vi "IsHotGoalDB.vi"(7 "Timeout (ms)":u32, 8 "error in":errorcluster, 9 "DBHot?":string="Boolean", 10 "DBFinished?":string="Boolean", 11 "DBStart":string="Boolean") -> (0 "error out":errorcluster, 1 "TimedOut?":bool, 2 "Hot?":bool, 3 "ElapsedTime":u32)   [LabVIEW 2015]
doc: "IsHotGoalDB determines whether or not the goal is hot. Image processing is done on the laptop (through the DB).\n-DBStart: the name of the DB boolean control that starts image processing. IsHotGoalDB writes to this to signal the DB to start.\n-DBFinished?: the name of the DB boolean indicator that indicates when the DB is done processing.\n-DBHot?: the name of the DB boolean indicator that indicates whether the goal is hot."
panel:
  in  "milliseconds to wait":u32=20
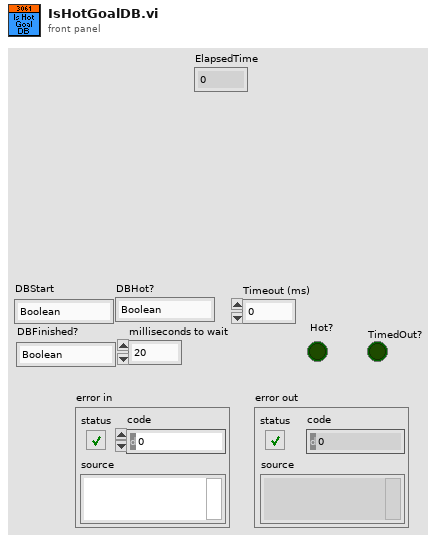
[diagram p1: front panel]
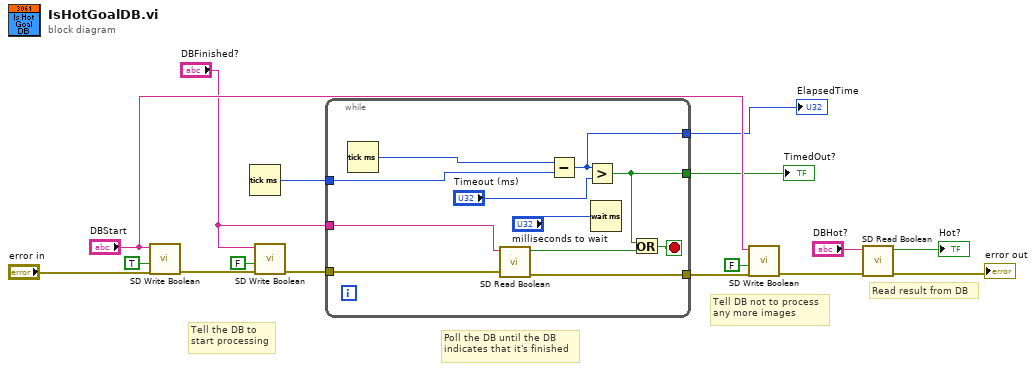
[diagram p0: block diagram]
diagram:
  # "Tell DB not to process\nany more images"
  # "Read result from DB"
  # "Poll the DB until the DB\nindicates that it's finished"
  # "Tell the DB to\nstart processing"
  n1 = call <vilib>:"SD Write Boolean.vi"("error in"="error in", "Boolean"=TRUE, "Name"="DBStart") -> ("error out"=w8:errorcluster)  [unwired: 7 in, 1 out]
  n2 = Tick Count (ms)() -> (millisecond timer value=w4:u32)
  n3 = call <vilib>:"SD Write Boolean.vi"("error in"=w8, "Boolean"=FALSE, "Name"="DBFinished?") -> ("error out"=w7:errorcluster)  [unwired: 7 in, 1 out]
  n4 = while {
    tunnel: w7 -> [w27]
    tunnel: [w26] -> w11
    tunnel: "DBFinished?" -> [w25]
    tunnel: w4 -> [w20]
    tunnel: [w18] -> w3
    tunnel: [w17] -> w1
    stop <- w23 stop-if-true
    n5 = Tick Count (ms)() -> (millisecond timer value=w21:u32)
    n6 = call <vilib>:"SD Read Boolean.vi"("error in"=w27, "Name"=w25) -> ("error out"=w26:errorcluster, "Boolean"=w22:bool)  [unwired: 7 in, 1 out]
    n7 = Subtract(x=w21, y=w20) -> (x-y=w17:u32)
    n8 = Greater?(x=w17, y="Timeout (ms)") -> (0:w18:bool)
    n9 = Wait (ms)(milliseconds to wait="milliseconds to wait") -> ()  [unwired: 1 out]
    n10 = Or(x=w18, y=w22) -> (x .or. y?=w23:bool)
  }
  "TimedOut?" <- w3
  "ElapsedTime" <- w1
  n11 = call <vilib>:"SD Write Boolean.vi"("error in"=w11, "Boolean"=FALSE, "Name"="DBStart") -> ("error out"=w10:errorcluster)  [unwired: 7 in, 1 out]
  n12 = call <vilib>:"SD Read Boolean.vi"("error in"=w10, "Name"="DBHot?") -> ("error out"=→"error out":errorcluster, "Boolean"=→"Hot?":bool)  [unwired: 7 in, 1 out]
